vi "Begin.vi"() -> (0 "error out":errorcluster)   [LabVIEW 2013]
doc: "Called before other user functions, this VI is expected to open initial I/O refnums, load in file data, and do all program initialization. Notice that the <B>error out</B> terminal is simply used for data flow. Wiring it to other structures or subVIs ensures that this VI runs first."
uses:
  <vilib>/Rock Robotics/WPI/DriverStation/WPI_DriverStationRobotMode2.ctl
  <vilib>/Rock Robotics/WPI/Joystick/WPI_JoystickDeviceEnum.ctl
  <vilib>/Rock Robotics/SystemInterfaces/DIO/FPGA_DIOPWMChannel.ctl
  <vilib>/Rock Robotics/SystemInterfaces/Typedef/FPGA_TypedefDigitalModule.ctl
  <vilib>/Rock Robotics/SystemInterfaces/DIO/FPGA_DIOChannel.ctl
  <vilib>/Rock Robotics/SystemInterfaces/AI/FPGA_AIChannel.ctl
  <vilib>/Rock Robotics/SystemInterfaces/Typedef/FPGA_TypedefAnalogModule.ctl
  Robot Global Data.vi
  <vilib>/Rock Robotics/WPI/MotorControl/WPI_MotorControlOpen Talon.vi
panel:
  out "error out 3":errorcluster
  out "error out 2":errorcluster
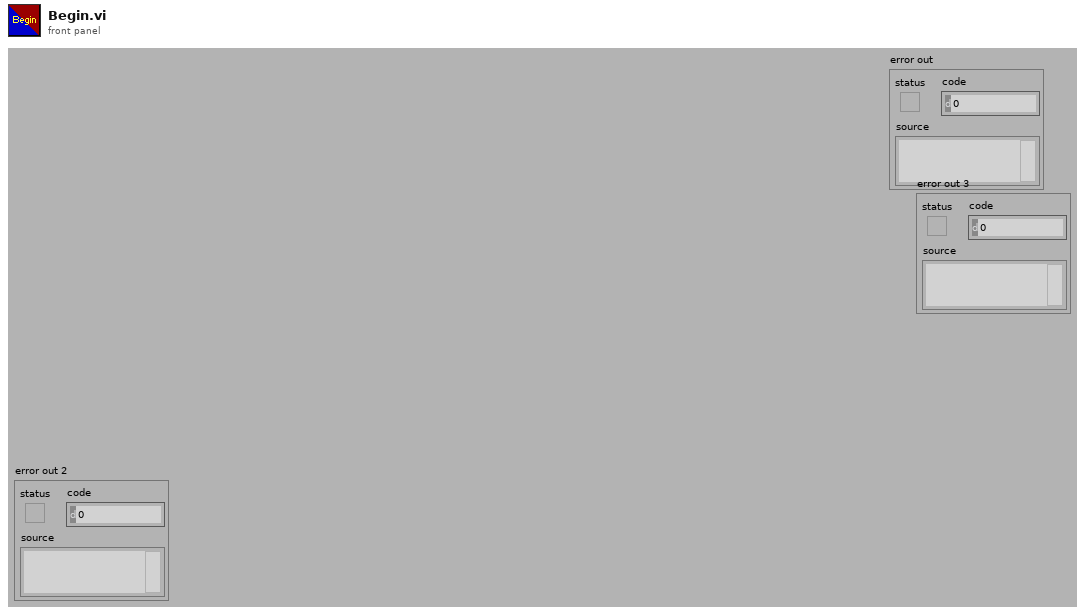
[diagram p1: front panel]
types:
  T1 = typedef "FPGA_DIOChannel.ctl" = enum8{"DIO 1", "DIO 2", "DIO 3", "DIO 4", "DIO 5", "DIO 6", "DIO 7", "DIO 8", "DIO 9", "DIO 10", "DIO 11", "DIO 12", "DIO 13", "DIO 14", "Invalid"}
  T2 = typedef "FPGA_TypedefDigitalModule.ctl" = enum16{"Digital Module 1", "Digital Module 2"}
  T3 = typedef "FPGA_DIOPWMChannel.ctl" = enum8{"PWM 1", "PWM 2", "PWM 3", "PWM 4", "PWM 5", "PWM 6", "PWM 7", "PWM 8", "PWM 9", "PWM 10", "Invalid"}
  T4 = typedef "FPGA_TypedefAnalogModule.ctl" = enum16{"Analog Module 1", "Analog Module 2"}
  T5 = typedef "FPGA_AIChannel.ctl" = enum8{"AI 1", "AI 2", "AI 3", "AI 4", "AI 5", "AI 6", "AI 7", "AI 8", "Invalid"}
  T6 = typedef "WPI_JoystickDeviceEnum.ctl" = enum16{"USB 1", "USB 2", "USB 3", "USB 4", "Kinect 1", "Kinect 2"}
  T7 = typedef "WPI_DriverStationRobotMode2.ctl" = enum16{"Autonomous Disabled", "Autonomous Enabled", "Teleop Disabled", "Teleop Enabled", "Timeout", "Finish", "Test Disabled", "Test Enabled"}
  T8 = typedef "WPI_JoystickDevRef.ctl" = cluster{"Device":T6}
  T9 = typedef "WPI_MotorControlDeviceRef.ctl" = cluster{"DeviceStatus":errorcluster, "Type":enum16{"PWM", "CAN"}, "PWM":cluster{"Digital Module":T2, "PWM Channel":T3, "DeadBand":T10}, "CAN":cluster{"Device Number":u8, "Control Mode":T11, "Semaphore":T12, "Max Vout":dbl}, "Invert":bool, "TransformRef":T13, "InvTransformRef":T13}
  T10 = typedef "WPI_PWMDeadband.ctl" = cluster{"Name":string, "maxPositivePwm":i32, "minPositivePwm":i32, "centerPwm":i32, "maxNegativePwm":i32, "minNegativePwm":i32, "angularRange":u16}
  T11 = typedef "WPI_CANJaguar_ControlMode.ctl" = enum8{"Percent VBus", "Current", "Speed", "Position", "Voltage"}
  T12 = typedef "Semaphore RefNum" = refnum<k1>
  T13 = typedef "WPI_PWMTransform_ConPane.ctl" = refnum<vi>
  T14 = typedef "WPI_ServoDeviceRef.ctl" = cluster{"DeviceStatus":errorcluster, "Digital Module":T2, "PWM Channel":T3, "DeadBand":T10}
  T15 = typedef "WPI_DigitalInputDevRef.ctl" = cluster{"DevStatus":errorcluster, "DIO Channel":T1, "Digital Module":T2}
  T16 = typedef "WPI_AnalogChannelDevRef.ctl" = cluster{"DevStatus":errorcluster, "Analog Module":T4, "Analog Channel":T5}
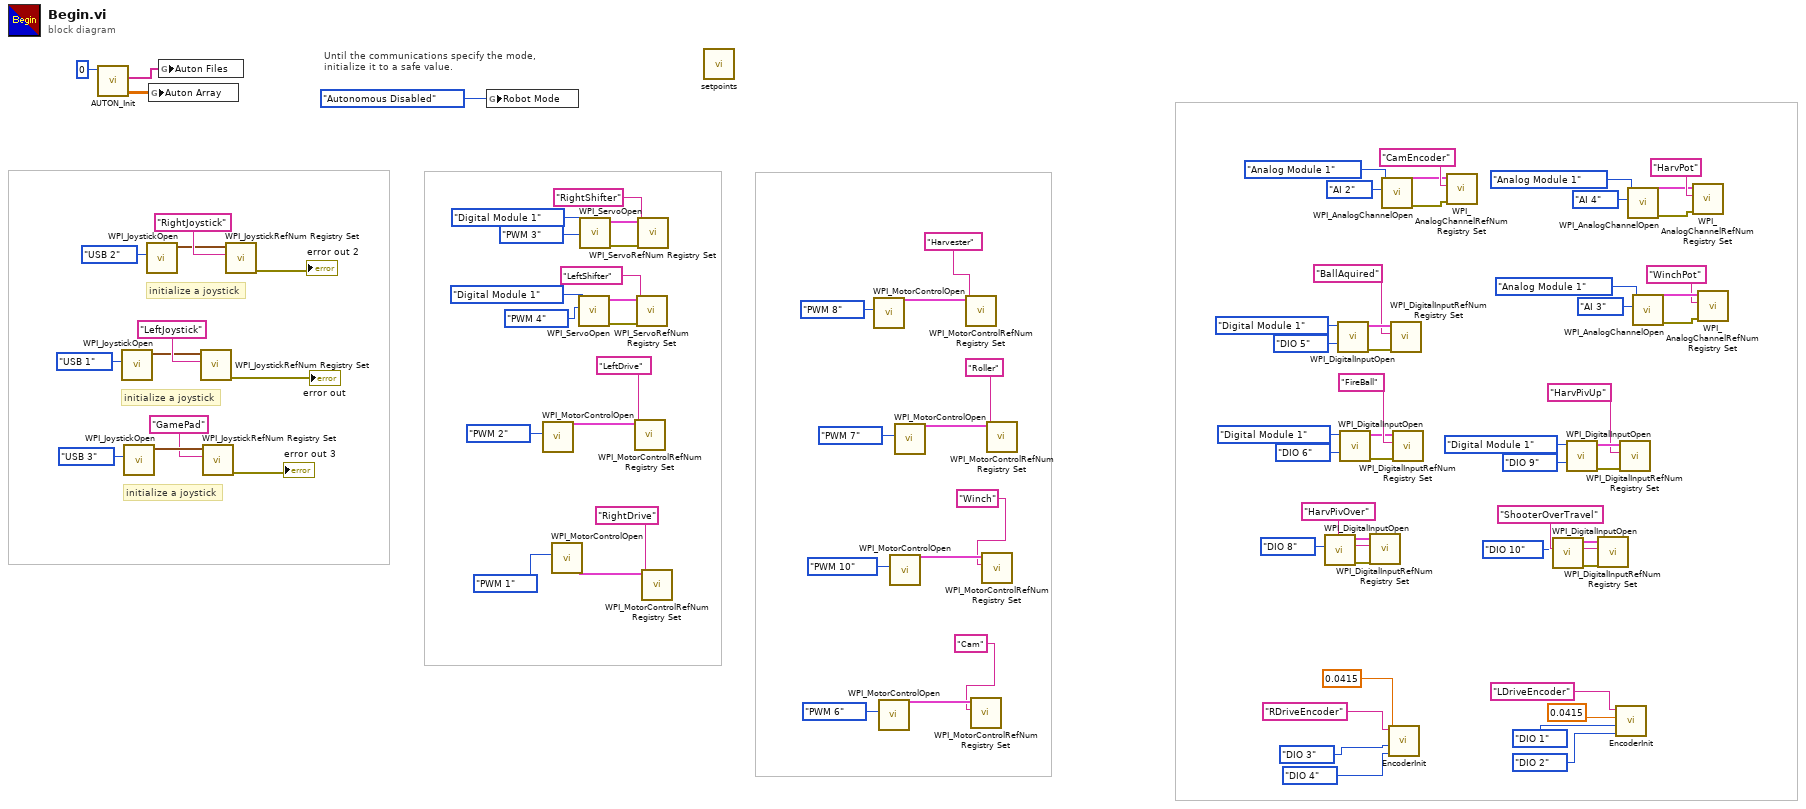
[diagram p0: block diagram]
diagram:
  # "initialize a joystick"
  # "initialize a joystick"
  # "initialize a joystick"
  # "Until the communications specify the mode,\ninitialize it to a safe value."
  n1 = call "AUTON_Init.vi"("Default File"=0) -> ("Auton Array"=w2:dbl[][], "Auton Files"=w1:string[])  [unwired: 8 in, 1 out]
  n2 = call <vilib>:"WPI_JoystickOpen.vi"("JoystickDevice"=WPI_JoystickDeviceEnum."USB 1") -> ("JoystickDevRef"=w88:T8)  [unwired: 10 in]
  n3 = call <vilib>:"WPI_JoystickOpen.vi"("JoystickDevice"=WPI_JoystickDeviceEnum."USB 3") -> ("JoystickDevRef"=w63:T8)  [unwired: 10 in]
  n4 = call <vilib>:"WPI_JoystickOpen.vi"("JoystickDevice"=WPI_JoystickDeviceEnum."USB 2") -> ("JoystickDevRef"=w84:T8)  [unwired: 10 in]
  n5 = global write "Robot Global Data.vi" "Auton Array"(w2) -> ()
  n6 = global write "Robot Global Data.vi" "Auton Files"(w1) -> ()
  n7 = call <vilib>:"WPI_JoystickRefNum Registry Set.vi"("refnum name"="LeftJoystick", "JoystickDevRef"=w88) -> ("error out"=→"error out":errorcluster)  [unwired: 8 in, 1 out]
  n8 = call <vilib>:"WPI_JoystickRefNum Registry Set.vi"("refnum name"="GamePad", "JoystickDevRef"=w63) -> ("error out"=→"error out 3":errorcluster)  [unwired: 8 in, 1 out]
  n9 = call <vilib>:"WPI_JoystickRefNum Registry Set.vi"("refnum name"="RightJoystick", "JoystickDevRef"=w84) -> ("error out"=→"error out 2":errorcluster)  [unwired: 8 in, 1 out]
  n10 = global write "Robot Global Data.vi" "Robot Mode"(WPI_DriverStationRobotMode2."Autonomous Disabled" ("Robot Mode")) -> ()
  n11 = call-poly <vilib>:"WPI_MotorControlOpen.vi"("PWM Channel"=FPGA_DIOPWMChannel."PWM 2") -> ("MotorControlDeviceRef"=w80:T9)  [unwired: 9 in, 1 out]
  n12 = call-poly <vilib>:"WPI_MotorControlOpen.vi"("PWM Channel"=FPGA_DIOPWMChannel."PWM 1") -> ("MotorControlDeviceRef"=w77:T9)  [unwired: 9 in, 1 out]
  n13 = call <vilib>:"WPI_ServoOpen.vi"("PWM Channel"=FPGA_DIOPWMChannel."PWM 4", "Digital Module (Module 1)"=FPGA_TypedefDigitalModule."Digital Module 1") -> ("error out"=w17:errorcluster, "ServoDeviceRef"=w10:T14)  [unwired: 8 in]
  n14 = call <vilib>:"WPI_ServoOpen.vi"("PWM Channel"=FPGA_DIOPWMChannel."PWM 3", "Digital Module (Module 1)"=FPGA_TypedefDigitalModule."Digital Module 1") -> ("error out"=w16:errorcluster, "ServoDeviceRef"=w15:T14)  [unwired: 8 in]
  n15 = call <vilib>:"WPI_MotorControlRefNum Registry Set.vi"("refnum name"="LeftDrive", "MotorControlDevRef"=w80) -> ()  [unwired: 8 in, 2 out]
  n16 = call <vilib>:"WPI_ServoRefNum Registry Set.vi"("error in (no error)"=w17, "refnum name"="LeftShifter", "ServoDeviceRef"=w10) -> ()  [unwired: 7 in, 2 out]
  n17 = call <vilib>:"WPI_ServoRefNum Registry Set.vi"("error in (no error)"=w16, "refnum name"="RightShifter", "ServoDeviceRef"=w15) -> ()  [unwired: 7 in, 2 out]
  n18 = call <vilib>:"WPI_MotorControlRefNum Registry Set.vi"("refnum name"="RightDrive", "MotorControlDevRef"=w77) -> ()  [unwired: 8 in, 2 out]
  n19 = call "setpoints.vi"() -> ()  [unwired: 12 in]
  n20 = call-poly <vilib>:"WPI_MotorControlOpen.vi"("PWM Channel"=FPGA_DIOPWMChannel."PWM 8") -> ("MotorControlDeviceRef"=w74:T9)  [unwired: 9 in, 1 out]
  n21 = call-poly <vilib>:"WPI_MotorControlOpen.vi"("PWM Channel"=FPGA_DIOPWMChannel."PWM 6") -> ("MotorControlDeviceRef"=w45:T9)  [unwired: 9 in, 1 out]
  n22 = call-poly <vilib>:"WPI_MotorControlOpen.vi"("PWM Channel"=FPGA_DIOPWMChannel."PWM 10") -> ("MotorControlDeviceRef"=w47:T9)  [unwired: 9 in, 1 out]
  n23 = call-poly <vilib>:"WPI_MotorControlOpen.vi"("PWM Channel"=FPGA_DIOPWMChannel."PWM 7") -> ("MotorControlDeviceRef"=w72:T9)  [unwired: 9 in, 1 out]
  n24 = call <vilib>:"WPI_MotorControlRefNum Registry Set.vi"("refnum name"="Harvester", "MotorControlDevRef"=w74) -> ()  [unwired: 8 in, 2 out]
  n25 = call <vilib>:"WPI_MotorControlRefNum Registry Set.vi"("refnum name"="Cam", "MotorControlDevRef"=w45) -> ()  [unwired: 8 in, 2 out]
  n26 = call <vilib>:"WPI_MotorControlRefNum Registry Set.vi"("refnum name"="Winch", "MotorControlDevRef"=w47) -> ()  [unwired: 8 in, 2 out]
  n27 = call <vilib>:"WPI_MotorControlRefNum Registry Set.vi"("refnum name"="Roller", "MotorControlDevRef"=w72) -> ()  [unwired: 8 in, 2 out]
  n28 = call <vilib>:"WPI_DigitalInputOpen.vi"("DIO Channel"=FPGA_DIOChannel."DIO 8") -> ("error out"=w49:errorcluster, "DigitalInputDevRef"=w50:T15)  [unwired: 9 in]
  n29 = call <vilib>:"WPI_DigitalInputOpen.vi"("DIO Channel"=FPGA_DIOChannel."DIO 5", "Digital Module (Module 1)"=FPGA_TypedefDigitalModule."Digital Module 1") -> ("error out"=w70:errorcluster, "DigitalInputDevRef"=w69:T15)  [unwired: 8 in]
  n30 = call <vilib>:"WPI_DigitalInputOpen.vi"("DIO Channel"=FPGA_DIOChannel."DIO 6", "Digital Module (Module 1)"=FPGA_TypedefDigitalModule."Digital Module 1") -> ("error out"=w33:errorcluster, "DigitalInputDevRef"=w34:T15)  [unwired: 8 in]
  n31 = call <vilib>:"WPI_DigitalInputRefNum Registry Set.vi"("error in (no error)"=w49, "refnum name"="HarvPivOver", "DigitalInputDevRef"=w50) -> ()  [unwired: 7 in, 2 out]
  n32 = call <vilib>:"WPI_AnalogChannelOpen.vi"("Analog Channel"=FPGA_AIChannel."AI 2", "Analog Module (Module 1)"=FPGA_TypedefAnalogModule."Analog Module 1") -> ("error out"=w39:errorcluster, "AIDeviceRef"=w38:T16)  [unwired: 8 in]
  n33 = call "EncoderInit.vi"("refnum name"="RDriveEncoder", "DistancePerCount"=0.0415, "DIO Channel"=FPGA_DIOChannel."DIO 3", "DIO Channel 2"=FPGA_DIOChannel."DIO 4") -> ()  [unwired: 7 in]
  n34 = call <vilib>:"WPI_DigitalInputRefNum Registry Set.vi"("error in (no error)"=w70, "refnum name"="BallAquired", "DigitalInputDevRef"=w69) -> ()  [unwired: 7 in, 2 out]
  n35 = call <vilib>:"WPI_DigitalInputRefNum Registry Set.vi"("error in (no error)"=w33, "refnum name"="FireBall", "DigitalInputDevRef"=w34) -> ()  [unwired: 7 in, 2 out]
  n36 = call <vilib>:"WPI_AnalogChannelRefNum Registry Set.vi"("error in (no error)"=w39, "refnum name"="CamEncoder", "AIDeviceRef"=w38) -> ()  [unwired: 7 in, 2 out]
  n37 = call <vilib>:"WPI_DigitalInputOpen.vi"("DIO Channel"=FPGA_DIOChannel."DIO 10") -> ("error out"=w7:errorcluster, "DigitalInputDevRef"=w6:T15)  [unwired: 9 in]
  n38 = call <vilib>:"WPI_DigitalInputOpen.vi"("DIO Channel"=FPGA_DIOChannel."DIO 9", "Digital Module (Module 1)"=FPGA_TypedefDigitalModule."Digital Module 1") -> ("error out"=w22:errorcluster, "DigitalInputDevRef"=w21:T15)  [unwired: 8 in]
  n39 = call <vilib>:"WPI_DigitalInputRefNum Registry Set.vi"("error in (no error)"=w7, "refnum name"="ShooterOverTravel", "DigitalInputDevRef"=w6) -> ()  [unwired: 7 in, 2 out]
  n40 = call "EncoderInit.vi"("refnum name"="LDriveEncoder", "DistancePerCount"=0.0415, "DIO Channel"=FPGA_DIOChannel."DIO 1", "DIO Channel 2"=FPGA_DIOChannel."DIO 2") -> ()  [unwired: 7 in]
  n41 = call <vilib>:"WPI_DigitalInputRefNum Registry Set.vi"("error in (no error)"=w22, "refnum name"="HarvPivUp", "DigitalInputDevRef"=w21) -> ()  [unwired: 7 in, 2 out]
  n42 = call <vilib>:"WPI_AnalogChannelOpen.vi"("Analog Channel"=FPGA_AIChannel."AI 4", "Analog Module (Module 1)"=FPGA_TypedefAnalogModule."Analog Module 1") -> ("error out"=w29:errorcluster, "AIDeviceRef"=w28:T16)  [unwired: 8 in]
  n43 = call <vilib>:"WPI_AnalogChannelOpen.vi"("Analog Channel"=FPGA_AIChannel."AI 3", "Analog Module (Module 1)"=FPGA_TypedefAnalogModule."Analog Module 1") -> ("error out"=w60:errorcluster, "AIDeviceRef"=w61:T16)  [unwired: 8 in]
  n44 = call <vilib>:"WPI_AnalogChannelRefNum Registry Set.vi"("error in (no error)"=w29, "refnum name"="HarvPot", "AIDeviceRef"=w28) -> ()  [unwired: 7 in, 2 out]
  n45 = call <vilib>:"WPI_AnalogChannelRefNum Registry Set.vi"("error in (no error)"=w60, "refnum name"="WinchPot", "AIDeviceRef"=w61) -> ()  [unwired: 7 in, 2 out]
